vi "F Dwf Analog Out Wait Info.vi"(7 "psecMax":dbl, 8 "error in (no error)":errorcluster, 9 "psecMin":dbl, 10 "idxChannel":i32, 11 "hdwf":i32) -> (0 "error out":errorcluster, 1 "psecMin out":dbl, 3 "function return":i32, 5 "psecMax out":dbl)   [LabVIEW 2021, in "Olasdwf.lvlib"]
doc: "DWFAPI int FDwfAnalogOutWaitInfo(HDWF hdwf, int idxChannel, double *psecMin, double *psecMax);"
uses:
  Olasdwf.lvlib
  Windows/System32/dwf.dll
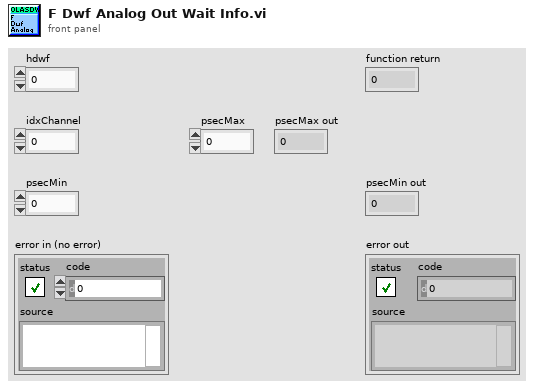
[diagram p1: front panel]
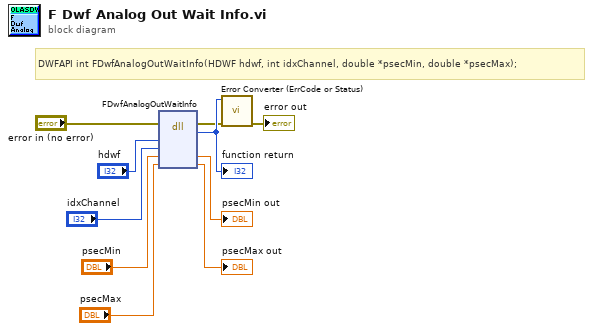
[diagram p0: block diagram]
diagram:
  # "DWFAPI int FDwfAnalogOutWaitInfo(HDWF hdwf, int idxChannel, double *psecMin, double *psecMax);"
  n1 = dll-call lib="/Windows/System32/dwf.*" fn="FDwfAnalogOutWaitInfo"(error in="error in (no error)", "hdwf"="hdwf", "idxChannel"="idxChannel", "psecMin"="psecMin", "psecMax"="psecMax") -> (error out=w2:errorcluster, w10:i32, "psecMin"=→"psecMin out":dbl, "psecMax"=→"psecMax out":dbl)  [unwired: 4 in, 1 out]
  "function return" <- w10
  n2 = call "Error Converter (ErrCode or Status).vi"("error in (no error)"=w2, "error code"=w10) -> ("error out"=→"error out":errorcluster)  [unwired: 9 in]
